vi "Set Alignment.vi"(8 "error in (no error)":errorcluster, 10 "Alignment":u16(ring)=1 items=["LEFT"=1, "CENTER"=2, "RIGHT"=3, "BOTH"=4, "MEDIUM_KASHIDA"=5, "DISTRIBUTE"=6, "NUM_TAB"=7, "HIGH_KASHIDA"=8, "LOW_KASHIDA"=9, "THAI_DISTRIBUTE"=10], 11 "xwpfParagraph in":refnum<class "xwpfParagraph.lvclass">) -> (0 "error out":errorcluster, 3 "xwpfParagraph out":refnum<class "xwpfParagraph.lvclass">)   [LabVIEW 2017, in "Word_Specific.lvlib" / "xwpfParagraph.lvclass"]
uses:
  xwpfParagraph.lvclass
  xwpfParagraph.lvclass/xwpfParagraph.ctl
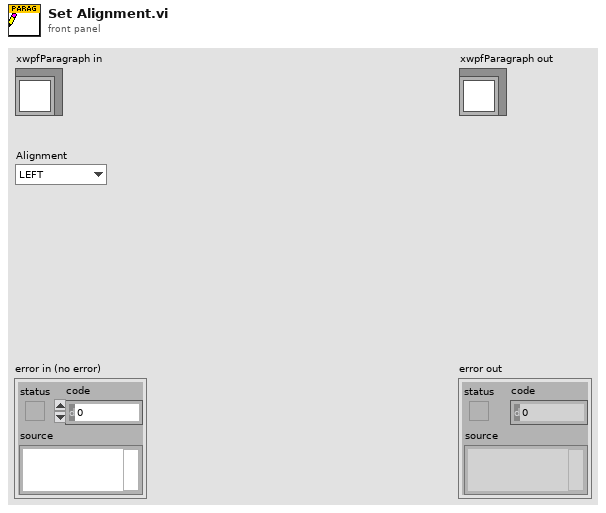
[diagram p1: front panel]
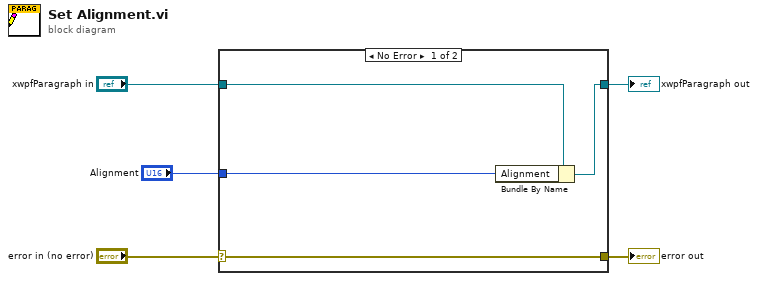
[diagram p0: block diagram]
diagram:
  n1 = case shown="No Error" "error in (no error)" {
    selector: "error in (no error)" -> [w9 w10]
    tunnel: [w9 w10] -> w4
    tunnel: [w7 w11] -> w2
    tunnel: "xwpfParagraph in" -> [w8 w11]
    tunnel: "Alignment" -> [w6 _]
    frame No Error {
      n2 = Bundle By Name(cluster=w8, "Alignment"=w6) -> (w7:refnum<class "xwpfParagraph.lvclass">)
    }
    frame Error {
    }
  }
  "error out" <- w4
  "xwpfParagraph out" <- w2
